vi "Stack2 (FGV).vi"(7 "Action":enum16{"Get", "Set Temp", "Set Fan"}(ring), 10 "Data Element":variant) -> (2 "Stack out":T1 {"Power-Setpoint" format="%d %"; "Purge Valve" scale=0.0..100.0; "Supply Valve" scale=0.0..100.0; "Switch" scale=0.0..100.0; "Voltage" format="%#.2f V"; "Current" format="%#.2f A"; "Pressure" format="%#.0f mbar"; "Thermometer" format="%#.1f °C"; "Fan" format="%d %"; "Power" format="%d W"})   [LabVIEW 2024]
uses:
  Stack.ctl
  Progress Bar Switch.ctl
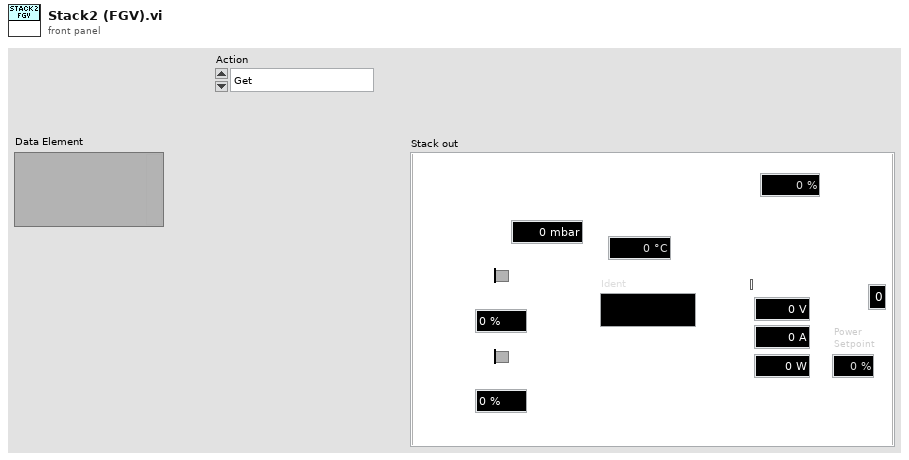
[diagram p1: front panel]
types:
  T1 = typedef "Stack.ctl" = cluster{"Ident":string, "Power":dbl, "Fan":dbl, "Thermometer":dbl, "MCU":u8, "Pressure":dbl, "Current":dbl, "Voltage":dbl, "Switch 2":bool, "Switch 3":bool, "Switch":T2, "Switch 4":bool, "Supply Valve":dbl, "Purge Valve":dbl, "Power-Setpoint":dbl}
  T2 = typedef "Progress Bar Switch.ctl" = u8
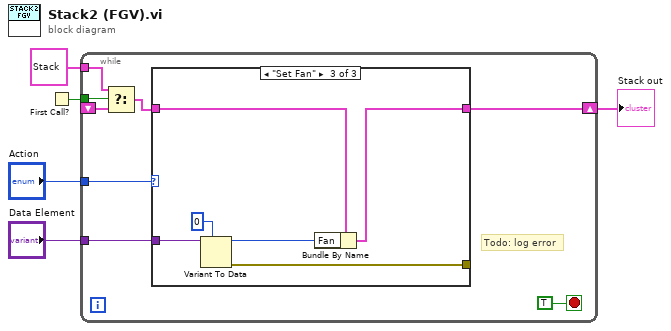
[diagram p0: block diagram]
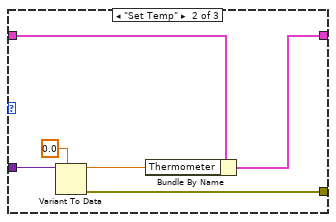
[diagram p3: hidden frame]
diagram:
  n1 = First Call?() -> (First Call?: T/F=w2:bool)
  n2 = while {
    shift-right: [w13] -> w3
    shift-left: _ -> [w8]
    tunnel: "Action" -> [w11]
    tunnel: "Data Element" -> [w10]
    tunnel: w2 -> [w9]
    tunnel: T1 {"Ident"="", "Power"=0.0, "Fan"=0.0, "Thermometer"=0.0, "MCU"=0, "Pressure"=0.0, "Current"=0.0, "Voltage"=0.0, "Switch 2"=FALSE, "Switch 3"=FALSE, "Switch"=0, "Switch 4"=FALSE, "Supply Valve"=0.0, "Purge Valve"=0.0, "Power-Setpoint"=0.0} ("Stack out") -> [w7]
    stop <- TRUE stop-if-true
    # "Todo: log error"
    n3 = Select(t=w7, s=w9, f=w8) -> (s? t:f=w6:T1)
    n4 = case shown="\"Set Fan\"" w11 {
      tunnel: [w14 w20 w22] -> w13
      tunnel: w6 -> [w14 w19 w25]
      tunnel: w10 -> [_ w18 w23]
      tunnel: [_ w15 w21] -> _
      frame "Get", Default {
      }
      frame "Set Temp" {
        n5 = Variant To Data(type=0.0, Variant=w18) -> (data=w17:dbl, error out=w15:errorcluster)  [unwired: 1 in]
        n6 = Bundle By Name(cluster=w19, "Thermometer"=w17) -> (w20:T1)
      }
      frame "Set Fan" {
        n7 = Variant To Data(type=u8 0, Variant=w23) -> (data=w24:u8, error out=w21:errorcluster)  [unwired: 1 in]
        n8 = Bundle By Name(cluster=w25, "Fan"=w24) -> (w22:T1)
      }
    }
  }
  "Stack out" <- w3
